vi "set_loop_end.vi"(9 "Loop Start Channel":i32, 10 "Input":T1) -> (2 "Output":T1)   [LabVIEW 2013]
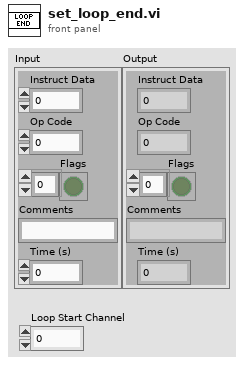
[diagram p1: front panel]
types:
  T1 = cluster{"Instruct Data":i32, "Op Code":i32, "Flags":bool[], "Comments":string, "Time (s)":dbl}
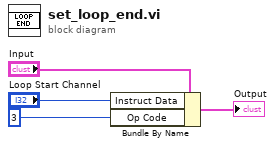
[diagram p0: block diagram]
diagram:
  n1 = Bundle By Name(cluster="Input", "Instruct Data"="Loop Start Channel", "Op Code"=3) -> (→"Output":T1)
